vi "Calculator Example.vi"() -> ()   [LabVIEW 2019, in "lv-classprovidershell-example.lvlib"]
uses:
  lv-classprovidershell-example.lvlib
  Shell/MathFunction.lvclass
  71c0a575-8996-4c86-9cee-e517d6c6022b.vi
  71c0a575-8996-4c86-9cee-e517d6c6022b.vi/37c9f98c-3050-4682-8746-e8c4a58c5728.vi
  71c0a575-8996-4c86-9cee-e517d6c6022b.vi/13a4f596-2347-4156-9567-e3b5667bb25e.vi
  71c0a575-8996-4c86-9cee-e517d6c6022b.vi/74390ab3-28c6-4983-b882-7c69ca936fc0.vi
  71c0a575-8996-4c86-9cee-e517d6c6022b.vi/890bbd91-a647-411d-b79d-707c95ce522e.vi
  71c0a575-8996-4c86-9cee-e517d6c6022b.vi/3db1b1aa-a5d9-4bec-b099-7f121fe235b0.vi
  71c0a575-8996-4c86-9cee-e517d6c6022b.vi/4cbaf643-bcd4-4fb7-897d-196ebea7ee23.vi
  src/_Support/__File Exists - Scalar__ogtk.vi
  src/_Support/__Strip Path Extension - String__ogtk.vi
  <vilib>/Utility/LVLibp/Get Exported File List.vi
  <vilib>/Utility/LVClass/Get LV Class Default Value.vi
  src/_Support/__Wait(ms) If Input Valid.vi
  <vilib>/Utility/libraryn.llb/Recursive File List.vi
  <vilib>/Utility/libraryn.llb/Check if File or Folder Exists.vi
  src/_Support/__Recursive File List with Exclude Option.vi
panel:
  in  "MathFunctionSelector":i32(ring) items=["Divide", "Multiply", "Add", "Subtract"]
  in  "Exit":bool
  in  "Calculate":bool
  out "f(x,y)":dbl
  in  "y":dbl
  in  "x":dbl
  # "Overview: The math functions of this calculator are loaded as plugins. \n\nInstructions: \n1. Run the VI.\n2. Specify the math function and click Calculate."
  # "="
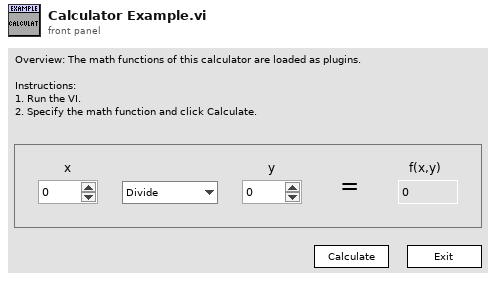
[diagram p1: front panel]
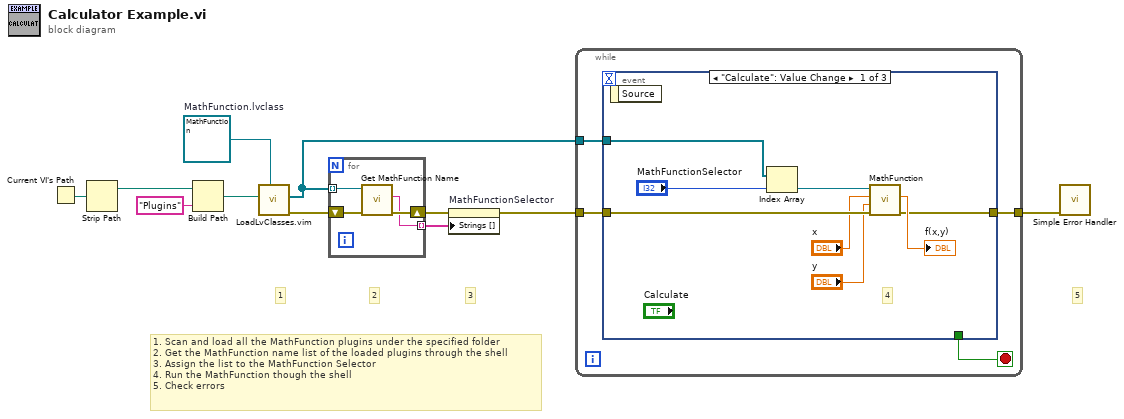
[diagram p0: block diagram]
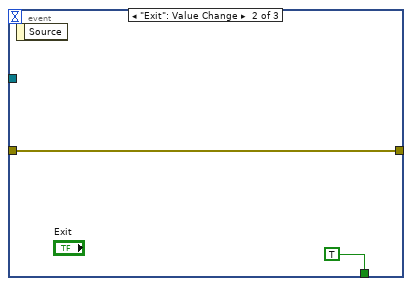
[diagram p2: hidden frame]
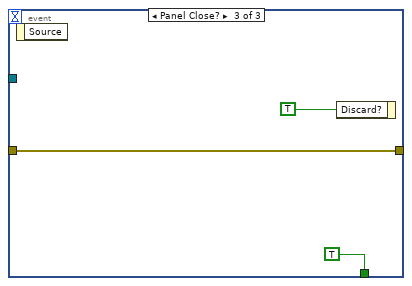
[diagram p3: hidden frame]
diagram:
  w1 = refnum<class "MathFunction.lvclass"> refnum  # MathFunction.lvclass
  # "1. Scan and load all the MathFunction plugins under the specified folder\n2. Get the MathFunction name list of the loaded plugins through the shell\n3. Assign the list to the MathFunction Selector\n4. Run the MathFunction though the shell\n5. Check errors"
  # "5"
  # "3"
  # "2"
  # "1"
  n1 = Current VI's Path() -> (path=w8:path)
  n2 = Strip Path(path=w8) -> (stripped path=w7:path)  [unwired: 1 out]
  n3 = Build Path(base path=w7, name or relative path="Plugins") -> (appended path=w10:path)
  n4 = call "LoadLvClasses.vim"("ClassType"=w1, "Path"=w10) -> ("error out"=w9:errorcluster, "Loaded Classes"=w2:refnum<class "MathFunction.lvclass">[])  [unwired: 8 in]
  n5 = for {
    tunnel: w2 -> [w15] mode=indexing
    shift-right: [w13] -> w6
    shift-left: w9 -> [w14]
    tunnel: [w12] -> w3 mode=indexing
    n6 = call-dynamic "Get MathFunction Name.vi"("error in (no error)"=w14, "Calculator in"=w15) -> ("error out"=w13:errorcluster, "MathFunction Name"=w12:string)  [unwired: 7 in, 1 out]
  }
  n7 = property on="MathFunctionSelector" class="Ring (strict)"(error in=w6, "Strings []"=w3) -> (error out=w5:errorcluster)  [unwired: 1 in, 1 out]
  n8 = while {
    tunnel: w5 -> [w19]
    tunnel: [w18] -> w4
    tunnel: w2 -> [w16]
    stop <- w17 stop-if-true
    n9 = event shown="[0] \"Calculate\": Value Change" {
      selector: _ -> [_ _ _]
      dyn-events: _ -> [_ _ _]
      timeout: _ -> [_ _ _]
      tunnel: w19 -> [w27 w29 w31]
      tunnel: [w23 w29 w31] -> w18
      tunnel: [_ TRUE TRUE] -> w17
      tunnel: w16 -> [w21 _ _]
      event "Calculate": Value Change {
        # "4"
        n10 = event-data() -> ()  [unwired: 1 in, 1 out]
        n11 = Index Array(array=w21, index="MathFunctionSelector") -> (element=w20:refnum<class "MathFunction.lvclass">)
        n12 = call-dynamic "MathFunction.vi"("error in (no error)"=w27, "y"="y", "x"="x", "Calculator in"=w20) -> ("error out"=w23:errorcluster, "f(x,y)"=→"f(x,y)":dbl)  [unwired: 5 in, 1 out]
      }
      event "Exit": Value Change {
        n13 = event-data() -> ()  [unwired: 1 in, 1 out]
      }
      event Panel Close? {
        n14 = event-data() -> ()  [unwired: 1 in, 1 out]
        n15 = event-data("Discard?"=TRUE) -> ()  [unwired: 1 in, 1 out]
      }
    }
  }
  n16 = call <vilib>:"Simple Error Handler.vi"("error in (no error)"=w4) -> ()  [unwired: 4 in, 5 out]
